vi "Point to Unit.vi"(3 "X point":sgl, 4 "Unit (default = mm)":T1=enum."mm") -> (9 "X unit":sgl)   [LabVIEW 2012]
uses:
  Controls/Unit.ctl
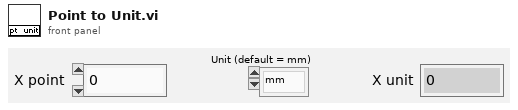
[diagram p1: front panel]
types:
  T1 = typedef "Unit.ctl" = enum16{"inch", "mm"}
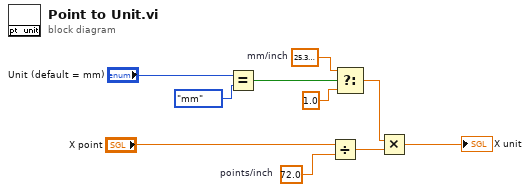
[diagram p0: block diagram]
diagram:
  w4 = sgl 25.4  # mm/inch
  w8 = sgl 72.0  # points/inch
  n1 = Equal?(x="Unit (default = mm)", y=Unit."mm") -> (x = y?=w5:bool)
  n2 = Divide(x="X point", y=w8) -> (x/y=w10:sgl)
  n3 = Select(t=w4, s=w5, f=sgl 1.0) -> (s? t:f=w1:sgl)
  n4 = Multiply(x=w1, y=w10) -> (x*y=→"X unit":sgl)
